vi "Connect.vi"(8 "error in":errorcluster, 11 "Thorlabs In":refnum<class "Thorlabs.lvclass">) -> (0 "error out":errorcluster, 3 "Thorlabs Out":refnum<class "Thorlabs.lvclass">)   [LabVIEW 2018, in "Thorlabs.lvlib" / "Thorlabs.lvclass"]
doc: "Override of the Connect.vi. This connects the actual Device up so that it can be used.\n\nCreator: Slade Jeppesen\nCreated: 09/29/2020"
uses:
  Thorlabs.lvclass
  Thorlabs.lvclass/Thorlabs.ctl
  C:/AME Test Engineering/LabVIEW/PPLs/Axis/DLLs/ThorLabs.MotionControl.KCube.DCServoCLI.dll
  PPLs/Axis/DLLs/ThorLabs.MotionControl.KCube.DCServoCLI.dll
  PPLs/Axis/Parent/Axis.lvlibp/Axis.lvclass
  C:/AME Test Engineering/LabVIEW/PPLs/Axis/Parent/Axis.lvlibp/Axis.lvclass
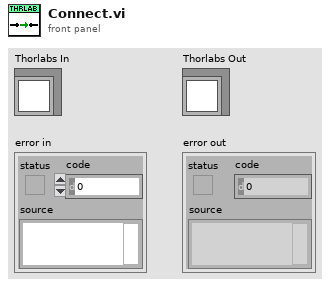
[diagram p1: front panel]
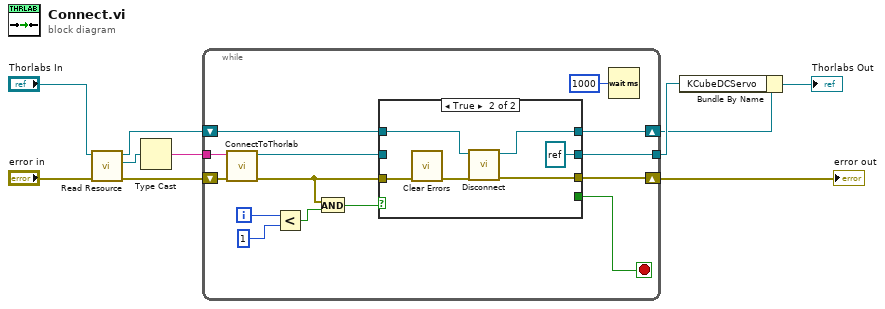
[diagram p0: block diagram]
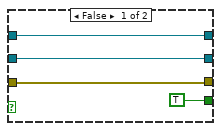
[diagram p2: hidden frame]
diagram:
  n1 = call "Read Resource.vi"("error in"="error in", "Axis in"="Thorlabs In") -> ("error out"=w3:errorcluster, "Resource"=w9:refnum<visa-resource-name>, "Axis out"=w2:refnum<class "Thorlabs.lvclass">)  [unwired: 7 in]
  n2 = Type Cast(x=w9) -> (*(type *) &x=w4:string)  [unwired: 1 in]
  n3 = while {
    tunnel: [w21] -> w6
    tunnel: w4 -> [w24]
    shift-right: [w18] -> w8
    shift-left: w3 -> [w23]
    shift-right: [w19] -> w1
    shift-left: w2 -> [w20]
    i -> [w13]
    stop <- w11 stop-if-true
    n4 = call "ConnectToThorlab.vi"("Error In"=w23, "Serial Number"=w24) -> ("Error Out"=w16:errorcluster, "KCubeDCServo"=w22:refnum<k24>)  [unwired: 8 in]
    n5 = Less?(x=w13, y=1) -> (x < y?=w14:bool)
    n6 = And(x=w16, y=w14) -> (x .and. y?=w15:bool)
    n7 = case shown="True" w15 {
      tunnel: w22 -> [w28 _]
      tunnel: [w28 refnum<k24> refnum ("KCubeDCServo")] -> w21
      tunnel: w20 -> [w27 w34]
      tunnel: [w27 w33] -> w19
      tunnel: [w26 w31] -> w18
      tunnel: w16 -> [w26 w29]
      tunnel: [TRUE _] -> w11
      frame False {
      }
      frame True {
        n8 = call <vilib>:"Clear Errors.vi"("error in (no error)"=w29) -> ("error out"=w32:errorcluster)  [unwired: 5 in, 1 out]
        n9 = call-dynamic "Disconnect.vi"("error in"=w32, "Thorlabs In"=w34) -> ("error out"=w31:errorcluster, "Thorlabs Out"=w33:refnum<class "Thorlabs.lvclass">)  [unwired: 8 in]
      }
    }
    n10 = Wait (ms)(milliseconds to wait=u32 1000) -> ()  [unwired: 1 out]
  }
  "error out" <- w8
  n11 = Bundle By Name(cluster=w1, "KCubeDCServo"=w6) -> (→"Thorlabs Out":refnum<class "Thorlabs.lvclass">)
